vi "Actor Last Ack.vi"(10 "Nested Actor":refnum<class "Actor.lvclass">, 11 "Self Actor in":refnum<class "Self Actor.lvclass">) -> (3 "Self Actor out":refnum<class "Self Actor.lvclass">)   [LabVIEW 2021, in "jettl.lvlib" / "Self Actor.lvclass"]
uses:
  Self Actor.lvclass
  Actor/Actor.lvclass
  Self Actor.lvclass/Self Actor.ctl
  jettl.lvlib
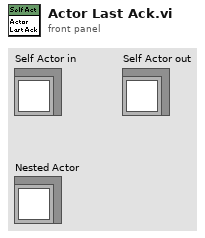
[diagram p1: front panel]
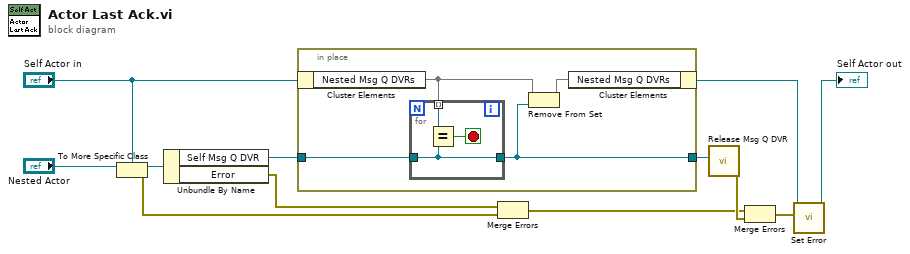
[diagram p0: block diagram]
diagram:
  n1 = To More Specific Class(target class="Self Actor in", reference="Nested Actor") -> (specific class reference=w12:refnum<class "Self Actor.lvclass">, error out=w1:errorcluster)  [unwired: 1 in]
  n2 = Unbundle By Name(w12) -> ("Self Msg Q DVR"=w10:refnum<data-value>, "Error"=w7:errorcluster)
  n3 = in-place {
    in-place-border: w10 -> [w14]
    in-place-border: [w13] -> w9
    n4 = in-place-cluster #1("Self Actor in") -> ("Nested Msg Q DVRs"=w16:set{refnum<data-value>})
    n5 = for {
      tunnel: w14 -> [w17]
      tunnel: w16 -> [w18] mode=indexing
      tunnel: [w17] -> w13
      stop <- w19 stop-if-true
      n6 = Equal?(x=w18, y=w17) -> (x = y?=w19:bool)
    }
    n7 = Remove From Set(10:w13, 11:w16) -> (3:w15:set{refnum<data-value>})  [unwired: 1 out]
    n8 = in-place-cluster #1("Nested Msg Q DVRs"=w15) -> (w6:refnum<class "Self Actor.lvclass">)
  }
  n9 = Merge Errors(w7, w1) -> (w2:errorcluster)
  n10 = call "Release Msg Q DVR.vi"("Msg Q DVR"=w9) -> ("error out"=w8:errorcluster)  [unwired: 10 in]
  n11 = Merge Errors(w2, w8) -> (w4:errorcluster)
  n12 = call-dynamic "Set Error.vi"("Error"=w4, "Self Actor in"=w6) -> ("Self Actor out"=→"Self Actor out":refnum<class "Self Actor.lvclass">)  [unwired: 9 in]
